vi "Write MSGLogger Message.vi"(8 "error in (no error)":errorcluster, 10 "Message to Log":refnum<class "MSG.lvclass">, 11 "MessageLoggerMessage in":refnum<class "MessageLoggerMessage.lvclass">) -> (0 "error out":errorcluster, 3 "MessageLoggerMessage out":refnum<class "MessageLoggerMessage.lvclass">)   [LabVIEW 2011, in "Messenging.lvlib" / "MessageLoggerMessage.lvclass"]
uses:
  MessageLoggerMessage.lvclass
  Interprocess Messenger/TextVarientMessage/MSG.lvclass
  MessageLoggerMessage.lvclass/MessageLoggerMessage.ctl
  <vilib>/regexp/Match Regular Expression.xnode
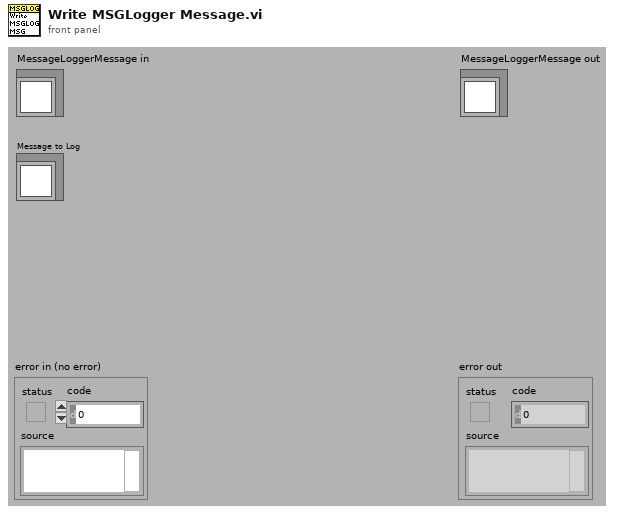
[diagram p1: front panel]
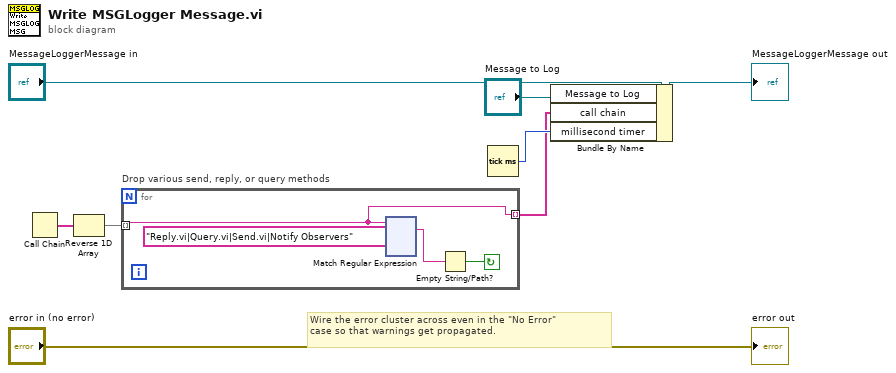
[diagram p0: block diagram]
diagram:
  # "Wire the error cluster across even in the \"No Error\"\ncase so that warnings get propagated."
  n1 = Call Chain() -> (call chain=w2:string[])
  n2 = Reverse 1D Array(array=w2) -> (reversed array=w1:string[])
  n3 = for "Drop various send, reply, or query methods" {
    tunnel: w1 -> [w9] mode=indexing
    tunnel: [w9] -> w3 mode=indexing
    stop <- w11 continue-if-true
    n4 = xnode "Match Regular Expression"("输入字符串"=w9, "正则表达式"="Reply.vi|Query.vi|Send.vi|Notify Observers" ("regular expression")) -> ("所有匹配"=w10:string)  [unwired: 3 in, 5 out]
    n5 = Empty String/Path?(string/path=w10) -> (empty?=w11:bool)
  }
  n6 = Tick Count (ms)() -> (millisecond timer value=w4:u32)
  n7 = Bundle By Name(cluster="MessageLoggerMessage in", "Message to Log"="Message to Log", "call chain"=w3, "millisecond timer"=w4) -> (→"MessageLoggerMessage out":refnum<class "MessageLoggerMessage.lvclass">)
  "error out" <- "error in (no error)"
